vi "Write Ver.vi"(10 "Ver":u8=1, 11 "SMSD ADU in":refnum<class "SMSD ADU.lvclass">) -> (3 "SMSD ADU out":refnum<class "SMSD ADU.lvclass">)   [LabVIEW 2021, in "SMSD ADU.lvclass"]
uses:
  SMSD ADU.lvclass
  SMSD ADU.lvclass/SMSD ADU.ctl
panel:
  out "error out":errorcluster
  in  "error in (no error)":errorcluster
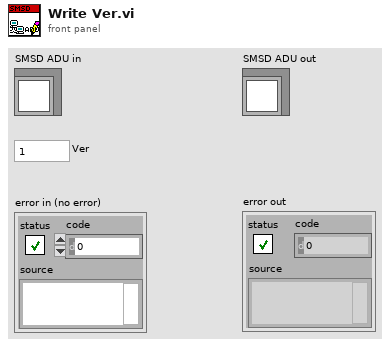
[diagram p1: front panel]
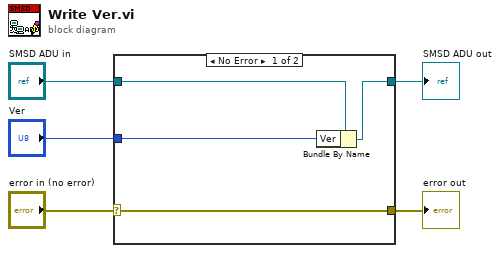
[diagram p0: block diagram]
diagram:
  n1 = case shown="No Error" "error in (no error)" {
    selector: "error in (no error)" -> [w6 w11]
    tunnel: "SMSD ADU in" -> [w9 w10]
    tunnel: [w8 w10] -> w4
    tunnel: "Ver" -> [w7 _]
    tunnel: [w6 w11] -> w1
    frame No Error {
      n2 = Bundle By Name(cluster=w9, "Ver"=w7) -> (w8:refnum<class "SMSD ADU.lvclass">)
    }
    frame Error {
    }
  }
  "SMSD ADU out" <- w4
  "error out" <- w1
